vi "PIL_ICR.vi"(8 "error in (no error)":errorcluster, 10 "ICR Queue":refnum<queue>, 11 "UI Queue":refnum<queue>) -> (0 "error out":errorcluster)   [LabVIEW 2024]
uses:
  controls/QMH_ICR_Message.ctl
  controls/QMH_ICR_Command.ctl
  controls/QMH_UI_Message.ctl
  controls/QMH_UI_Command.ctl
  controls/HARDWARE_Resources.ctl
  controls/PROCESSING_Inputs.ctl
  controls/OPO_Inputs.ctl
  controls/QMH_ICR_Cluster.ctl
panel:
  out "RF Trap is ON":bool=TRUE caption="RF Trap"
  in  "OPO Inputs":T1={"OPO AutoAlignment ON"=FALSE, "OPO Start Value"=210.0, "OPO Stop Value"=270.0, "OPO Step"=10.0} {"OPO Step" min=1.0 max=60.0; "OPO Stop Value" min=210.0 max=270.0; "OPO Start Value" min=210.0 max=270.0}
  out "Number of  Loops":i16
  out "Loop":i16
  out "Number of Excitations":i16 caption="Excitations"
  out "PROCESSING  Inputs":T2={"Reference Mass"=300.0939, "Cyclotron Freq"=255.727, "Magnetron Freq"=0.001} caption="DATA Inputs" {"Magnetron Freq" format="%.5g"; "Cyclotron Freq" format="%.5g"; "Reference Mass" format="%.5g"}
  in  "Start":bool
  in  "Stop":bool
  in  "Send Trigger":bool
  out "Total Duration":i32
  out "Number of  Accumulations":i16
  out "Accumulation":i16
  in  "Use Software Trigger":bool=TRUE
  in  "Graph Chooser":T3(radio)=enum."Mass Spectrum"
  out "Remaining Time":string
  out "Spectrum Path":path
  out "Spectrum Prefix":string
  out "Spectrum Name":string
  out "Accum Name":string
  out "Mass Accumulated":cluster{dbl[], dbl[]}(graph)
  out "Mass Spectrum":cluster{dbl[], dbl[]}(graph)
  out "Frequency Spectrum":cluster{dbl[], dbl[]}(graph)
  out "Signal":cluster{dbl[], dbl[]}(graph)
  in  "HARDWARE Resources":T4={"AO6711 Physical Channels"="Analog/ao0:3", "AO6711 Task Name"="", "AO_6738 Physical Channels"="AO_6738/ao0:3", "AO6738 Task Name"="", "AWG5421 Resource Name"="Waveform", "DIGIT 5122 Resource Name"="Digitizer", "HSDIO Resource Name"="Sequencer"}
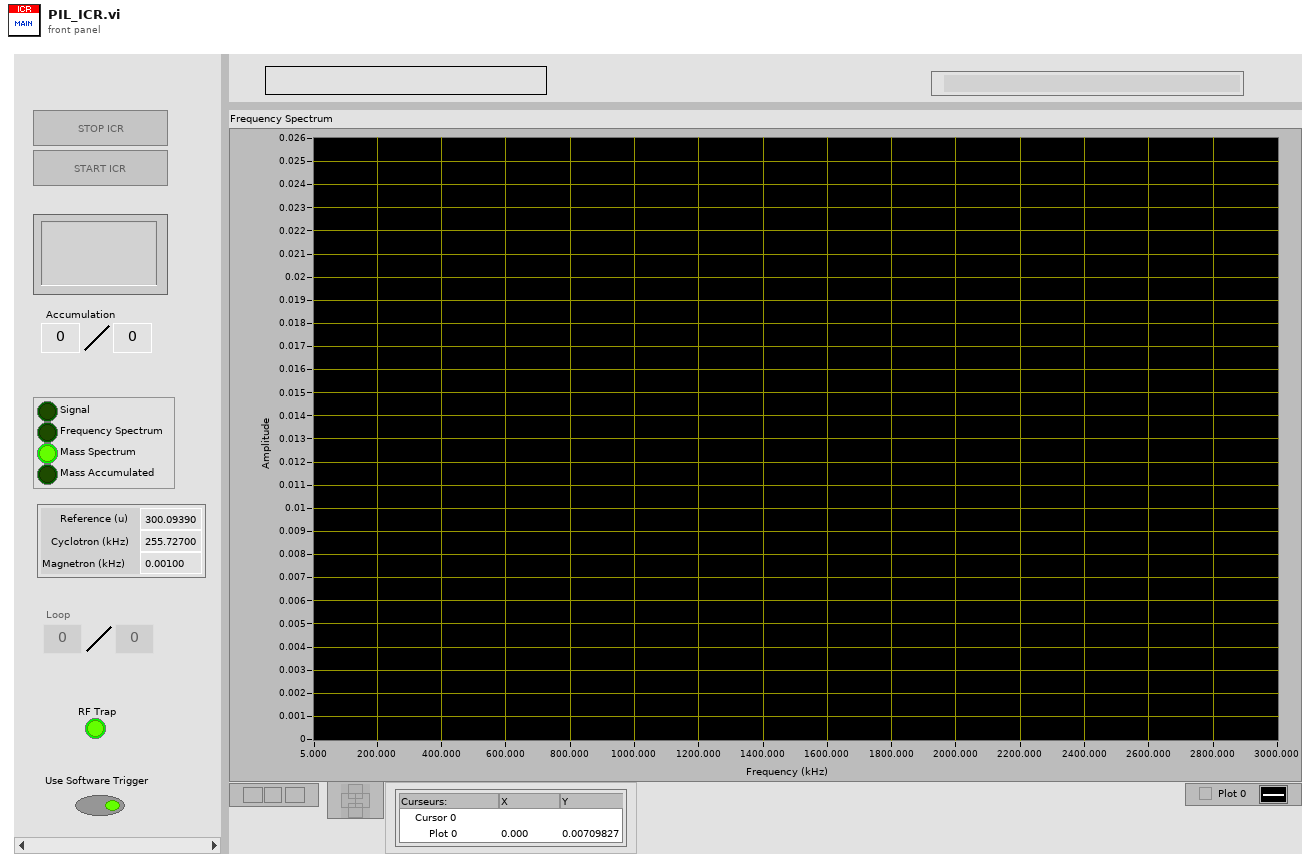
[diagram p1: front panel]
types:
  T1 = typedef "OPO_Inputs.ctl" = cluster{"OPO AutoAlignment ON":bool, "OPO Start Value":dbl, "OPO Stop Value":dbl, "OPO Step":dbl}
  T2 = typedef "PROCESSING_Inputs.ctl" = cluster{"Reference Mass":dbl, "Cyclotron Freq":dbl, "Magnetron Freq":dbl}
  T3 = enum32{"Signal", "Frequency Spectrum", "Mass Spectrum", "Mass Accumulated"}
  T4 = typedef "HARDWARE_Resources.ctl" = cluster{"AO6711 Physical Channels":tag, "AO6711 Task Name":refnum<k21>, "AO_6738 Physical Channels":tag, "AO6738 Task Name":refnum<k21>, "AWG5421 Resource Name":refnum<k15>, "DIGIT 5122 Resource Name":refnum<k15>, "HSDIO Resource Name":refnum<k15>}
  T5 = typedef "QMH_ICR_Cluster.ctl" = cluster{"Use Software Trigger":refnum<vi>, "Send Trigger":refnum<vi>, "Stop":refnum<vi>, "Start":refnum<vi>, "HARDWARE Resources":refnum<vi>, "Total Duration":refnum<vi>, "Remaining Time":refnum<vi>, "Accumulation":refnum<vi>, "Number of  Accumulations":refnum<vi>, "Number of  Excitations":refnum<vi>, "Graph Chooser":refnum<vi>, "Signal":refnum<vi>, "Frequency Spectrum":refnum<vi>, "Mass Spectrum":refnum<vi>, "Mass Accumulated":refnum<vi>, "Processing":refnum<vi>, "Spectrum Path":refnum<vi>, "Spectrum Prefix":refnum<vi>, "Spectrum Name":refnum<vi>, "Accum Name":refnum<vi>, "Disk Writing Done":refnum<notifier>, "Loop":refnum<vi>, "Number of Loops":refnum<vi>, "OPO Inputs":refnum<vi>, "RF Trap is ON":refnum<vi>}
  T6 = typedef "QMH_ICR_Command.ctl" = enum16{"Initialize", "Sequence Loop Setup", "Sequence Setup", "ICR Start", "ICR Stop", "Hardware Setup", "Next Sequence Loop", "Next Accumulation", "Waiting for Trigger", "Sequence Started", "Sequence Finished", "Sequence Loop Done", "Writing Data", "Hardware Reset", "Exit"}
  T7 = typedef "QMH_UI_Command.ctl" = enum16{"Initialize", "UI Load", "UI Save", "UI Save As", "UI Change Experiment", "UI Change Voltages", "UI Change Sequence", "UI Change Expert", "UI Change Loops", "UI Change Scientist", "Ready to Start", "UI Start", "Waiting for ICR", "UI Exit", "Update Experiment", "Update Report", "Update ICR Status", "Waiting for User"}
  T8 = typedef "QMH_ICR_Message.ctl" = cluster{"Command":T6, "Data":variant}
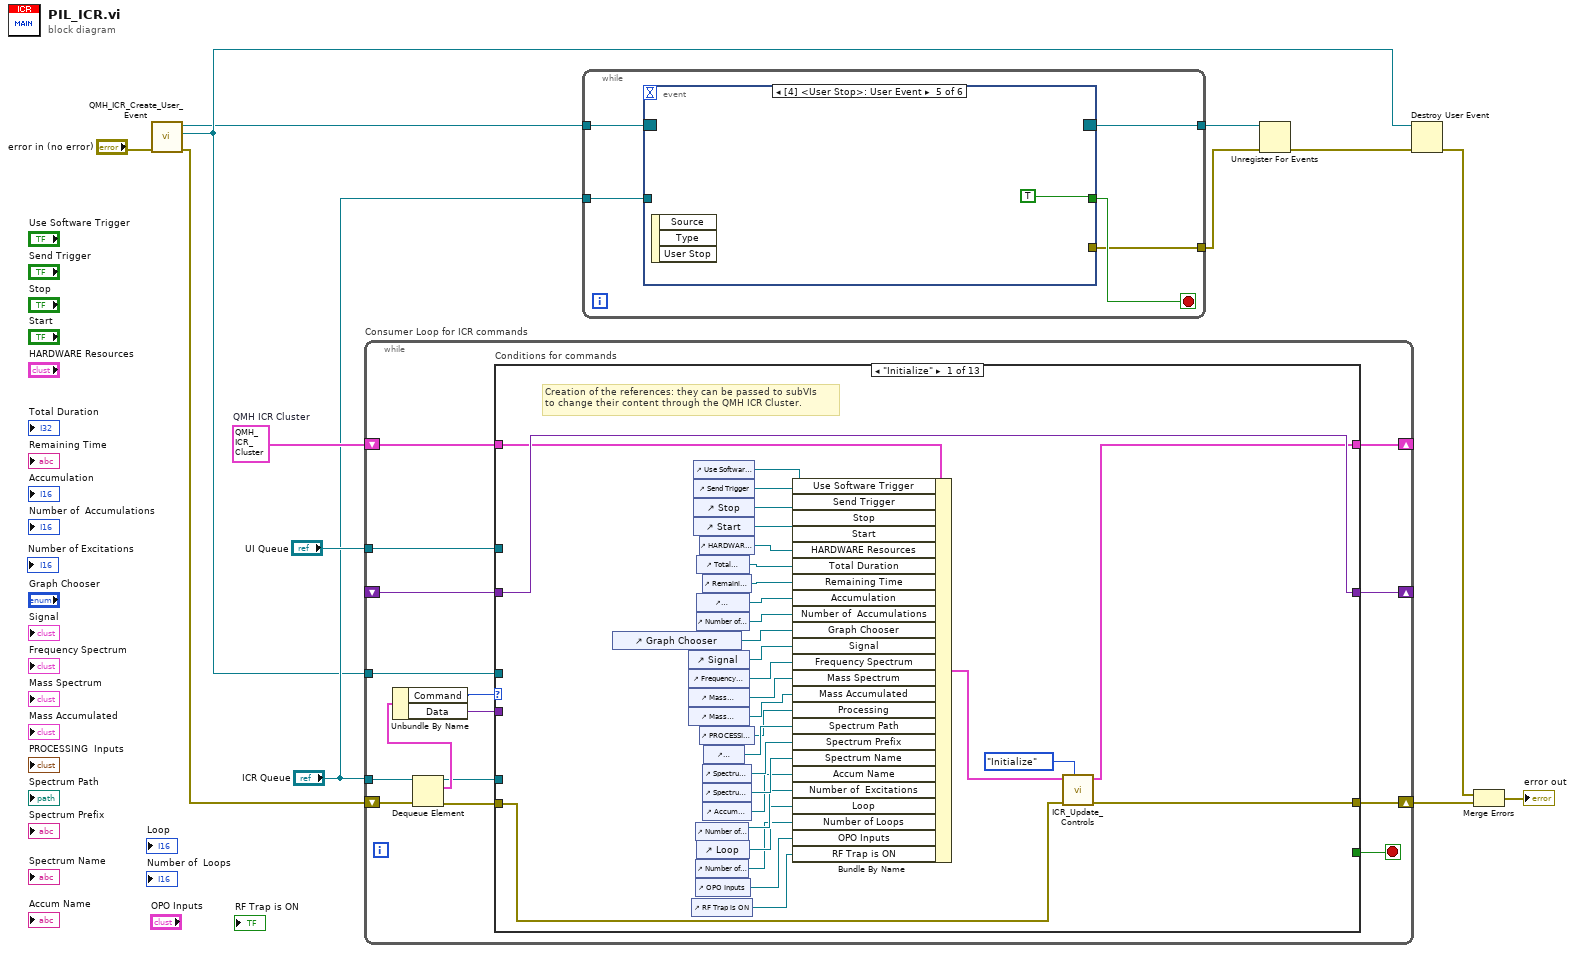
[diagram p0: block diagram]
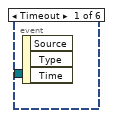
[diagram p2: hidden frame]
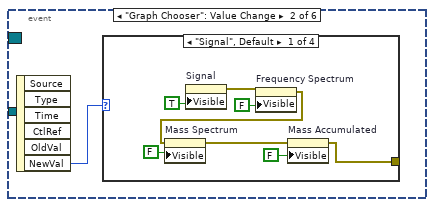
[diagram p3: hidden frame]
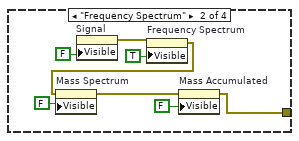
[diagram p4: hidden frame]
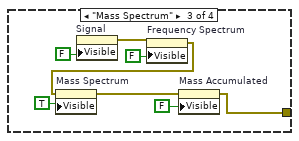
[diagram p5: hidden frame]
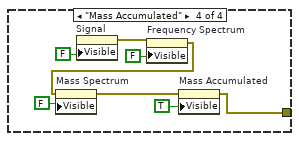
[diagram p6: hidden frame]
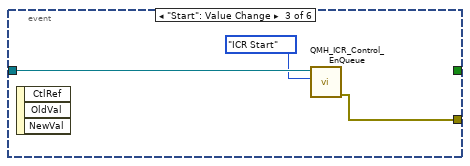
[diagram p7: hidden frame]
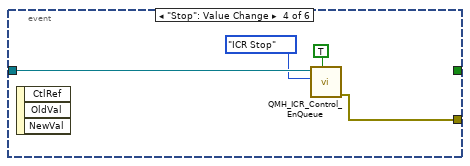
[diagram p8: hidden frame]
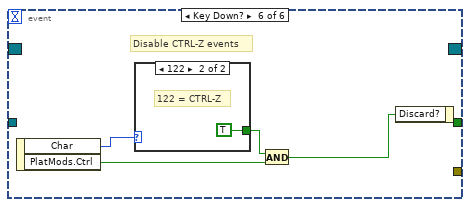
[diagram p9: hidden frame]
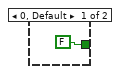
[diagram p10: hidden frame]
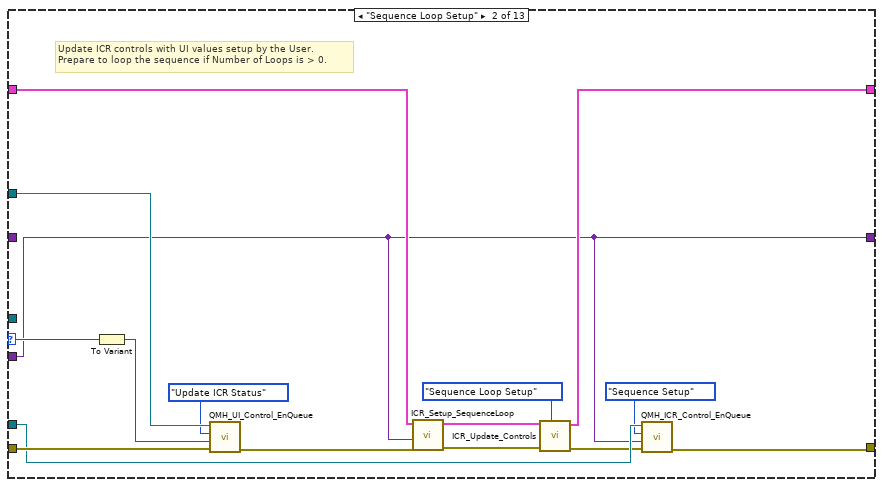
[diagram p11: hidden frame]
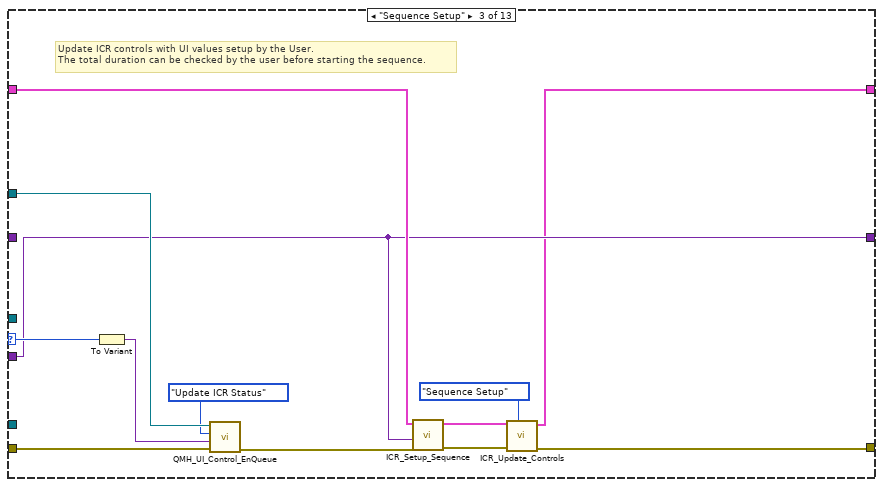
[diagram p12: hidden frame]
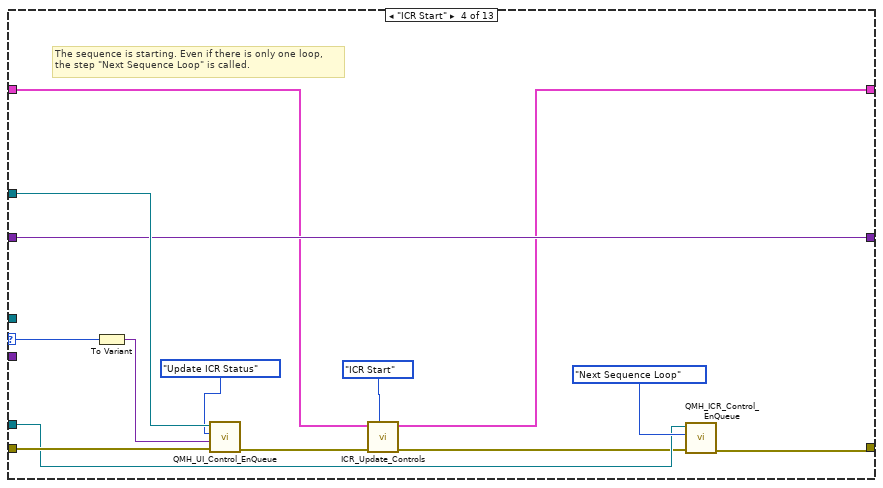
[diagram p13: hidden frame]
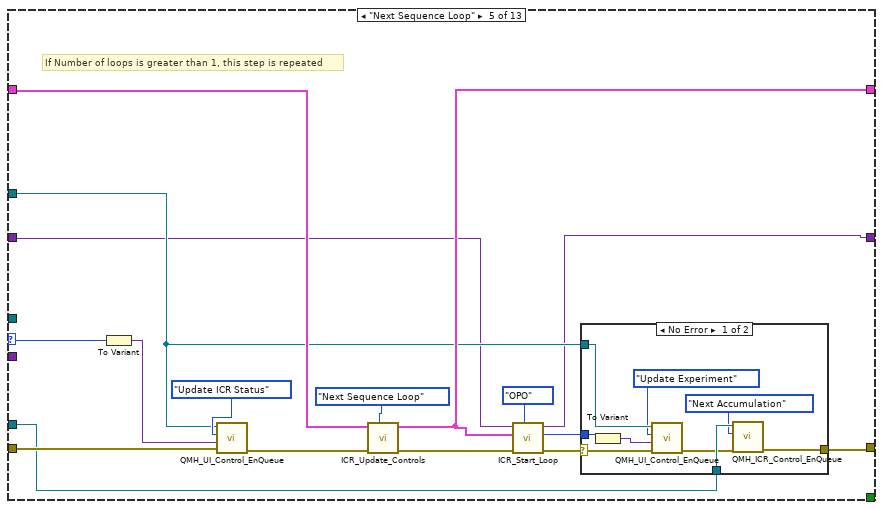
[diagram p14: hidden frame]
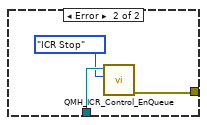
[diagram p15: hidden frame]
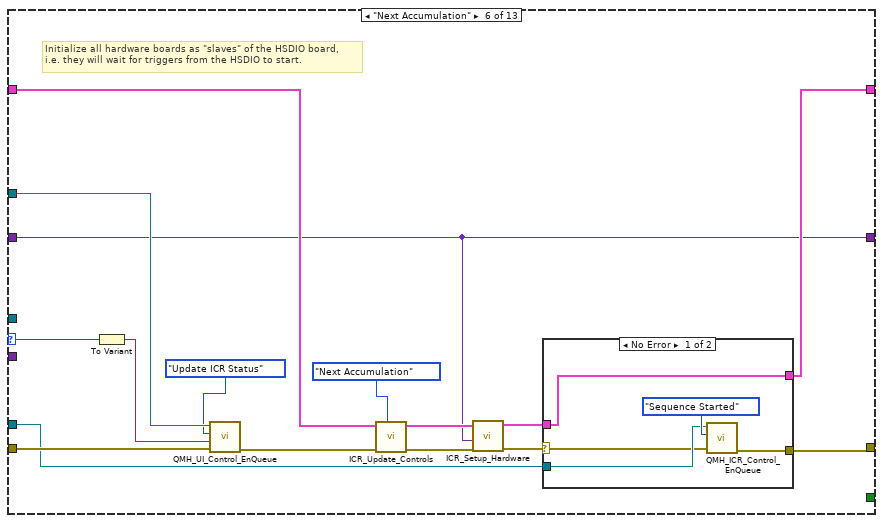
[diagram p16: hidden frame]
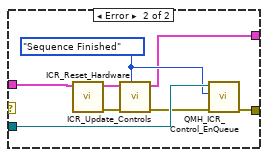
[diagram p17: hidden frame]
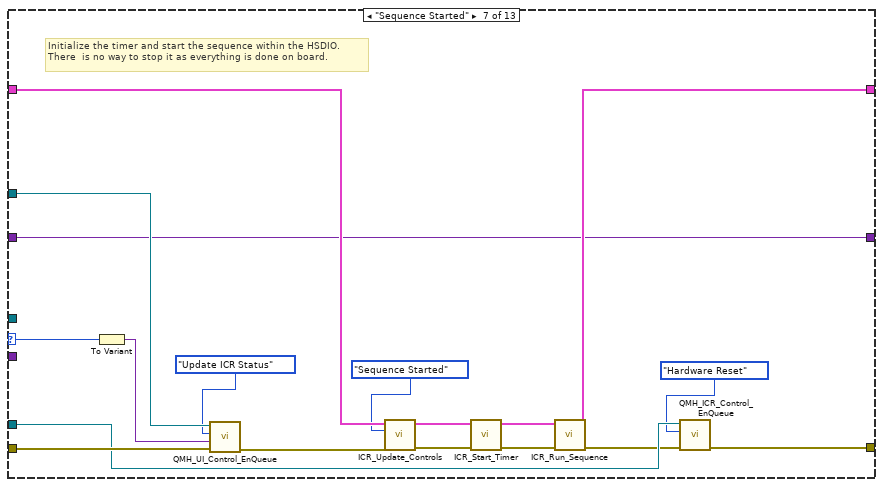
[diagram p18: hidden frame]
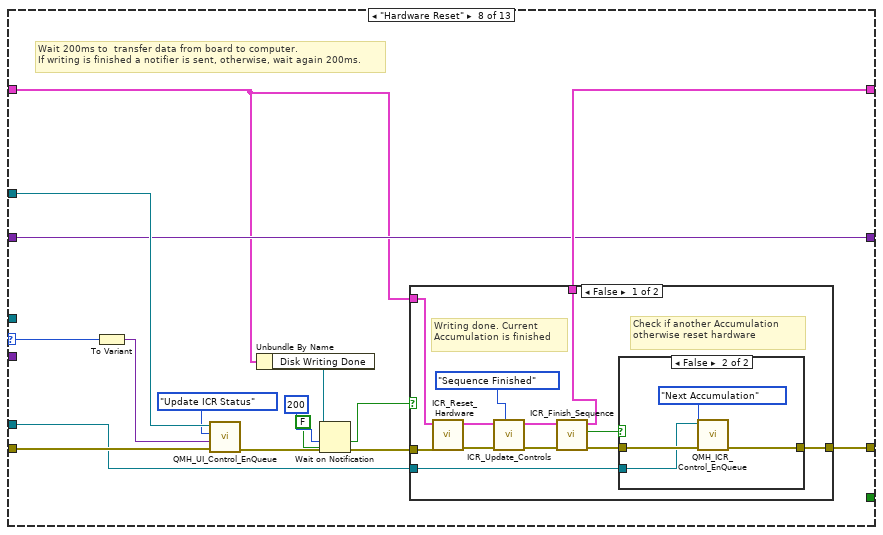
[diagram p19: hidden frame]
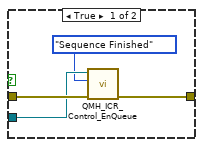
[diagram p20: hidden frame]
diagram:
  w6 = T5 {"Use Software Trigger"=refnum, "Send Trigger"=refnum, "Stop"=refnum, "Start"=refnum, "HARDWARE Resources"=refnum, "Total Duration"=refnum, "Remaining Time"=refnum, "Accumulation"=refnum, "Number of  Accumulations"=refnum, "Number of  Excitations"=refnum, "Graph Chooser"=refnum, "Signal"=refnum, "Frequency Spectrum"=refnum, "Mass Spectrum"=refnum, "Mass Accumulated"=refnum, "Processing"=refnum, "Spectrum Path"=refnum, "Spectrum Prefix"=refnum, "Spectrum Name"=refnum, "Accum Name"=refnum, "Disk Writing Done"=refnum, "Loop"=refnum, "Number of Loops"=refnum, "OPO Inputs"=refnum, "RF Trap is ON"=refnum}  # QMH ICR Cluster
  n1 = call "QMH_ICR_Create_User_Event.vi"("error in (no error)"="error in (no error)") -> ("error out"=w11:errorcluster, "User Stop Event"=w2:refnum<user-event>, "Refnum register for events"=w1:refnum<event-registration>)  [unwired: 8 in]
  n2 = while "Consumer Loop for ICR commands" {
    shift-right: [w19] -> w7
    shift-left: w11 -> [w26]
    tunnel: "ICR Queue" -> [w27]
    tunnel: "UI Queue" -> [w21]
    shift-right: [w18] -> _
    shift-left: _ -> [w17]
    tunnel: w2 -> [w16]
    shift-right: [w14] -> _
    shift-left: w6 -> [w15]
    stop <- w20 stop-if-true
    n3 = Dequeue Element(queue=w27, error in (no error)=w26) -> (queue out=w25:refnum<queue>, element=w28:T8, error out=w22:errorcluster)  [unwired: 2 out]
    n4 = Unbundle By Name(w28) -> ("Command"=w24:T6, "Data"=w23:variant)
    n5 = case "Conditions for commands" shown="\"Initialize\"" w24 {
      selector: w24 -> [_ w73 w86 w100 w114 w145 w176 w192 w234 w251 w277 _ _]
      tunnel: w25 -> [_ w64 _ w96 w111 w142 w173 w189 w228 w238 _ w287 _]
      tunnel: w23 -> [_ w60 w82 _ _ _ _ _ _ _ _ _ _]
      tunnel: w22 -> [w54 w72 w85 w99 w113 w144 w175 w191 w233 w250 w276 w279 _]
      tunnel: w21 -> [_ w74 w87 w101 w106 w146 w177 w193 w235 w252 w267 _ _]
      tunnel: [_ _ _ _ _ _ _ _ _ _ _ TRUE _] -> w20
      tunnel: [w52 w62 w77 w97 w116 w143 w174 w190 w230 w247 w275 w280 _] -> w19
      tunnel: [w59 w60 w82 w95 w104 w132 w169 w187 w232 w237 w274 _ _] -> w18
      tunnel: w17 -> [w59 _ _ w95 w105 w132 w169 w187 w232 w237 w274 _ _]
      tunnel: w16 -> [_ _ _ _ _ _ _ _ _ _ _ w284 _]
      tunnel: w15 -> [w51 w70 w83 w93 w112 w139 w172 w186 w225 w242 w272 _ _]
      tunnel: [w53 w67 w79 w92 w108 w135 w170 w188 w223 w244 w270 _ _] -> w14
      frame "Initialize" {
        # "Creation of the references: they can be passed to subVIs\nto change their content through the QMH ICR Cluster."
        n6 = control-ref of="Graph Chooser"() -> (w55:refnum<vi>)
        n7 = control-ref of="Signal"() -> (w34:refnum<vi>)
        n8 = control-ref of="Frequency Spectrum"() -> (w56:refnum<vi>)
        n9 = control-ref of="Mass Spectrum"() -> (w57:refnum<vi>)
        n10 = control-ref of="Mass Accumulated"() -> (w45:refnum<vi>)
        n11 = control-ref of="RF Trap is ON"() -> (w29:refnum<vi>)
        n12 = control-ref of="Use Software Trigger"() -> (w58:refnum<vi>)
        n13 = control-ref of="Send Trigger"() -> (w43:refnum<vi>)
        n14 = control-ref of="Stop"() -> (w42:refnum<vi>)
        n15 = control-ref of="Start"() -> (w41:refnum<vi>)
        n16 = control-ref of="Number of Excitations"() -> (w33:refnum<vi>)
        n17 = control-ref of="Number of  Loops"() -> (w31:refnum<vi>)
        n18 = control-ref of="OPO Inputs"() -> (w30:refnum<vi>)
        n19 = control-ref of="Total Duration"() -> (w39:refnum<vi>)
        n20 = control-ref of="Accumulation"() -> (w36:refnum<vi>)
        n21 = control-ref of="Number of  Accumulations"() -> (w35:refnum<vi>)
        n22 = control-ref of="Loop"() -> (w32:refnum<vi>)
        n23 = control-ref of="HARDWARE Resources"() -> (w40:refnum<vi>)
        n24 = control-ref of="PROCESSING  Inputs"() -> (w44:refnum<vi>)
        n25 = control-ref of="Remaining Time"() -> (w38:refnum<vi>)
        n26 = control-ref of="Spectrum Prefix"() -> (w47:refnum<vi>)
        n27 = control-ref of="Spectrum Name"() -> (w46:refnum<vi>)
        n28 = control-ref of="Accum Name"() -> (w37:refnum<vi>)
        n29 = control-ref of="Spectrum Path"() -> (w48:refnum<vi>)
        n30 = Bundle By Name(cluster=w51, "Use Software Trigger"=w58, "Send Trigger"=w43, "Stop"=w42, "Start"=w41, "HARDWARE Resources"=w40, "Total Duration"=w39, "Remaining Time"=w38, "Accumulation"=w36, "Number of  Accumulations"=w35, "Graph Chooser"=w55, "Signal"=w34, "Frequency Spectrum"=w56, "Mass Spectrum"=w57, "Mass Accumulated"=w45, "Processing"=w44, "Spectrum Path"=w48, "Spectrum Prefix"=w47, "Spectrum Name"=w46, "Accum Name"=w37, "Number of  Excitations"=w33, "Loop"=w32, "Number of Loops"=w31, "OPO Inputs"=w30, "RF Trap is ON"=w29) -> (w50:T5)
        n31 = call "ICR_Update_Controls.vi"("Command"=QMH_ICR_Command."Initialize", "error in (no error)"=w54, "QMH ICR Cluster"=w50) -> ("error out"=w52:errorcluster, "QMH ICR Cluster"=w53:T5)  [unwired: 7 in]
      }
      frame "Sequence Loop Setup" {
        # "Update ICR controls with UI values setup by the User.\nPrepare to loop the sequence if Number of Loops is > 0."
        n32 = To Variant(anything=w73) -> (Variant=w75:variant)
        n33 = call "QMH_UI_Control_EnQueue.vi"("error in (no error)"=w72, "Variant"=w75, "Command"=QMH_UI_Command."Update ICR Status", "UI Queue"=w74) -> ("error out"=w71:errorcluster)  [unwired: 6 in, 1 out]
        n34 = call "ICR_Setup_SequenceLoop.vi"("error in (no error)"=w71, "QMH UI Cluster"=w60, "QMH ICR Cluster"=w70) -> ("error out"=w69:errorcluster, "QMH ICR Cluster"=w68:T5)  [unwired: 7 in]
        n35 = call "ICR_Update_Controls.vi"("Command"=QMH_ICR_Command."Sequence Loop Setup", "error in (no error)"=w69, "QMH ICR Cluster"=w68) -> ("error out"=w63:errorcluster, "QMH ICR Cluster"=w67:T5)  [unwired: 7 in]
        n36 = call "QMH_ICR_Control_EnQueue.vi"("error in (no error)"=w63, "Variant"=w60, "Command"=QMH_ICR_Command."Sequence Setup", "ICR Queue"=w64) -> ("error out"=w62:errorcluster)  [unwired: 6 in, 1 out]
      }
      frame "Sequence Setup" {
        # "Update ICR controls with UI values setup by the User.\nThe total duration can be checked by the user before starting the sequence."
        n37 = To Variant(anything=w86) -> (Variant=w88:variant)
        n38 = call "QMH_UI_Control_EnQueue.vi"("error in (no error)"=w85, "Variant"=w88, "Command"=QMH_UI_Command."Update ICR Status", "UI Queue"=w87) -> ("error out"=w84:errorcluster)  [unwired: 6 in, 1 out]
        n39 = call "ICR_Setup_Sequence.vi"("error in (no error)"=w84, "QMH UI Cluster"=w82, "QMH ICR Cluster"=w83) -> ("error out"=w81:errorcluster, "QMH ICR Cluster"=w80:T5)  [unwired: 7 in]
        n40 = call "ICR_Update_Controls.vi"("Command"=QMH_ICR_Command."Sequence Setup", "error in (no error)"=w81, "QMH ICR Cluster"=w80) -> ("error out"=w77:errorcluster, "QMH ICR Cluster"=w79:T5)  [unwired: 7 in]
      }
      frame "ICR Start" {
        # "The sequence is starting. Even if there is only one loop,\nthe step \"Next Sequence Loop\" is called."
        n41 = To Variant(anything=w100) -> (Variant=w102:variant)
        n42 = call "QMH_UI_Control_EnQueue.vi"("error in (no error)"=w99, "Variant"=w102, "Command"=QMH_UI_Command."Update ICR Status", "UI Queue"=w101) -> ("error out"=w89:errorcluster)  [unwired: 6 in, 1 out]
        n43 = call "ICR_Update_Controls.vi"("Command"=QMH_ICR_Command."ICR Start", "error in (no error)"=w89, "QMH ICR Cluster"=w93) -> ("error out"=w90:errorcluster, "QMH ICR Cluster"=w92:T5)  [unwired: 7 in]
        n44 = call "QMH_ICR_Control_EnQueue.vi"("error in (no error)"=w90, "Command"=QMH_ICR_Command."Next Sequence Loop", "ICR Queue"=w96) -> ("error out"=w97:errorcluster)  [unwired: 7 in, 1 out]
      }
      frame "Next Sequence Loop" {
        # "If Number of loops is greater than 1, this step is repeated"
        n45 = To Variant(anything=w114) -> (Variant=w119:variant)
        n46 = call "QMH_UI_Control_EnQueue.vi"("error in (no error)"=w113, "Variant"=w119, "Command"=QMH_UI_Command."Update ICR Status", "UI Queue"=w106) -> ("error out"=w118:errorcluster)  [unwired: 6 in, 1 out]
        n47 = call "ICR_Update_Controls.vi"("Command"=QMH_ICR_Command."Next Sequence Loop", "error in (no error)"=w118, "QMH ICR Cluster"=w112) -> ("error out"=w110:errorcluster, "QMH ICR Cluster"=w108:T5)  [unwired: 7 in]
        n48 = call "ICR_Start_Loop.vi"("Loop Selector"=enum16{"OPO", "Other"}."OPO", "error in (no error)"=w110, "QMH ICR Cluster"=w108, "QMH UI Cluster"=w105) -> ("error out"=w103:errorcluster, "Loop Current Value"=w107:i16, "QMH UI Cluster Output"=w104:variant)  [unwired: 5 in]
        n49 = case shown="No Error" w103 {
          selector: w103 -> [w120 _]
          tunnel: [w128 w131] -> w116
          tunnel: w111 -> [w127 w130]
          tunnel: w107 -> [w124 _]
          tunnel: w106 -> [w122 _]
          frame No Error {
            n50 = To Variant(anything=w124) -> (Variant=w123:variant)
            n51 = call "QMH_UI_Control_EnQueue.vi"("error in (no error)"=w120, "Variant"=w123, "Command"=QMH_UI_Command."Update Experiment", "UI Queue"=w122) -> ("error out"=w125:errorcluster)  [unwired: 6 in, 1 out]
            n52 = call "QMH_ICR_Control_EnQueue.vi"("error in (no error)"=w125, "Command"=QMH_ICR_Command."Next Accumulation", "ICR Queue"=w127) -> ("error out"=w128:errorcluster)  [unwired: 7 in, 1 out]
          }
          frame Error {
            n53 = call "QMH_ICR_Control_EnQueue.vi"("Command"=QMH_ICR_Command."ICR Stop", "ICR Queue"=w130) -> ("error out"=w131:errorcluster)  [unwired: 8 in, 1 out]
          }
        }
      }
      frame "Next Accumulation" {
        # "Initialize all hardware boards as \"slaves\" of the HSDIO board,\ni.e. they will wait for triggers from the HSDIO to start."
        n54 = To Variant(anything=w145) -> (Variant=w147:variant)
        n55 = call "QMH_UI_Control_EnQueue.vi"("error in (no error)"=w144, "Variant"=w147, "Command"=QMH_UI_Command."Update ICR Status", "UI Queue"=w146) -> ("error out"=w141:errorcluster)  [unwired: 6 in, 1 out]
        n56 = call "ICR_Update_Controls.vi"("Command"=QMH_ICR_Command."Next Accumulation", "error in (no error)"=w141, "QMH ICR Cluster"=w139) -> ("error out"=w140:errorcluster, "QMH ICR Cluster"=w138:T5)  [unwired: 7 in]
        n57 = call "ICR_Setup_Hardware.vi"("error in (no error)"=w140, "QMH UI Cluster"=w132, "QMH ICR Cluster"=w138) -> ("error out"=w134:errorcluster, "QMH ICR Cluster"=w137:T5)  [unwired: 7 in]
        n58 = case shown="No Error" w134 {
          selector: w134 -> [w148 _]
          tunnel: [w151 w156] -> w143
          tunnel: w142 -> [w150 w158]
          tunnel: w137 -> [w149 w154]
          tunnel: [w149 w153] -> w135
          frame No Error {
            n59 = call "QMH_ICR_Control_EnQueue.vi"("error in (no error)"=w148, "Command"=QMH_ICR_Command."Sequence Started", "ICR Queue"=w150) -> ("error out"=w151:errorcluster)  [unwired: 7 in, 1 out]
          }
          frame Error {
            w155 = QMH_ICR_Command."Sequence Finished" ("Command")
            n60 = call "ICR_Reset_Hardware.vi"("QMH ICR Cluster"=w154) -> ("error out"=w159:errorcluster, "QMH ICR Cluster"=w160:T5)  [unwired: 9 in]
            n61 = call "ICR_Update_Controls.vi"("Command"=w155, "error in (no error)"=w159, "QMH ICR Cluster"=w160) -> ("error out"=w157:errorcluster, "QMH ICR Cluster"=w153:T5)  [unwired: 7 in]
            n62 = call "QMH_ICR_Control_EnQueue.vi"("error in (no error)"=w157, "Command"=w155, "ICR Queue"=w158) -> ("error out"=w156:errorcluster)  [unwired: 7 in, 1 out]
          }
        }
      }
      frame "Sequence Started" {
        # "Initialize the timer and start the sequence within the HSDIO. \nThere  is no way to stop it as everything is done on board."
        n63 = To Variant(anything=w176) -> (Variant=w178:variant)
        n64 = call "QMH_UI_Control_EnQueue.vi"("error in (no error)"=w175, "Variant"=w178, "Command"=QMH_UI_Command."Update ICR Status", "UI Queue"=w177) -> ("error out"=w166:errorcluster)  [unwired: 6 in, 1 out]
        n65 = call "ICR_Update_Controls.vi"("Command"=QMH_ICR_Command."Sequence Started", "error in (no error)"=w166, "QMH ICR Cluster"=w172) -> ("error out"=w163:errorcluster, "QMH ICR Cluster"=w167:T5)  [unwired: 7 in]
        n66 = call "ICR_Start_Timer.vi"("error in (no error)"=w163, "QMH ICR Cluster"=w167) -> ("error out"=w162:errorcluster, "QMH ICR Cluster"=w164:T5)  [unwired: 8 in]
        n67 = call "ICR_Run_Sequence.vi"("error in (no error)"=w162, "QMH ICR Cluster"=w164) -> ("error out"=w171:errorcluster, "QMH ICR Cluster"=w170:T5)  [unwired: 8 in]
        n68 = call "QMH_ICR_Control_EnQueue.vi"("error in (no error)"=w171, "Command"=QMH_ICR_Command."Hardware Reset", "ICR Queue"=w173) -> ("error out"=w174:errorcluster)  [unwired: 7 in, 1 out]
      }
      frame "Hardware Reset" {
        # "Wait 200ms to  transfer data from board to computer.\nIf writing is finished a notifier is sent, otherwise, wait again 200ms."
        n69 = To Variant(anything=w192) -> (Variant=w194:variant)
        n70 = call "QMH_UI_Control_EnQueue.vi"("error in (no error)"=w191, "Variant"=w194, "Command"=QMH_UI_Command."Update ICR Status", "UI Queue"=w193) -> ("error out"=w183:errorcluster)  [unwired: 6 in, 1 out]
        n71 = Unbundle By Name(w186) -> ("Disk Writing Done"=w185:refnum<notifier>)
        n72 = Wait on Notification(notifier=w185, ignore previous (F)=FALSE ("ignorer les précédents (F)"), timeout in ms (-1)=200 ("timeout en ms (-1)"), error in (no error)=w183) -> (timed out?=w181:bool, error out=w182:errorcluster)  [unwired: 2 out]
        n73 = case shown="False" w181 {
          tunnel: [w206 w220] -> w190
          tunnel: w189 -> [w205 w221]
          tunnel: [w203 w216] -> w188
          tunnel: w186 -> [w196 w217]
          tunnel: w182 -> [w195 w219]
          frame False {
            # "Check if another Accumulation\notherwise reset hardware"
            # "Writing done. Current \nAccumulation is finished"
            n74 = call "ICR_Reset_Hardware.vi"("error in (no error)"=w195, "QMH ICR Cluster"=w196) -> ("error out"=w199:errorcluster, "QMH ICR Cluster"=w201:T5)  [unwired: 8 in]
            n75 = call "ICR_Update_Controls.vi"("Command"=QMH_ICR_Command."Sequence Finished", "error in (no error)"=w199, "QMH ICR Cluster"=w201) -> ("error out"=w198:errorcluster, "QMH ICR Cluster"=w200:T5)  [unwired: 7 in]
            n76 = call "ICR_Finish_Sequence.vi"("error in (no error)"=w198, "QMH ICR Cluster"=w200) -> ("error out"=w204:errorcluster, "Is Finished ?"=w202:bool, "QMH ICR Cluster"=w203:T5)  [unwired: 7 in]
            n77 = case shown="False" w202 {
              tunnel: w204 -> [w210 w214]
              tunnel: [w209 w213] -> w206
              tunnel: w205 -> [w208 w212]
              frame True {
                n78 = call "QMH_ICR_Control_EnQueue.vi"("error in (no error)"=w210, "Command"=QMH_ICR_Command."Sequence Finished", "ICR Queue"=w208) -> ("error out"=w209:errorcluster)  [unwired: 7 in, 1 out]
              }
              frame False {
                n79 = call "QMH_ICR_Control_EnQueue.vi"("error in (no error)"=w214, "Command"=QMH_ICR_Command."Next Accumulation", "ICR Queue"=w212) -> ("error out"=w213:errorcluster)  [unwired: 7 in, 1 out]
              }
            }
          }
          frame True {
            # "Writing not done. Wait again by sending\nthe same message  to the ICR Queue"
            n80 = call "ICR_Update_Controls.vi"("Command"=QMH_ICR_Command."Hardware Reset", "error in (no error)"=w219, "QMH ICR Cluster"=w217) -> ("error out"=w218:errorcluster, "QMH ICR Cluster"=w216:T5)  [unwired: 7 in]
            n81 = call "QMH_ICR_Control_EnQueue.vi"("error in (no error)"=w218, "Command"=QMH_ICR_Command."Hardware Reset", "ICR Queue"=w221) -> ("error out"=w220:errorcluster)  [unwired: 7 in, 1 out]
          }
        }
      }
      frame "Sequence Finished" {
        n82 = To Variant(anything=w234) -> (Variant=w236:variant)
        n83 = call "QMH_UI_Control_EnQueue.vi"("error in (no error)"=w233, "Variant"=w236, "Command"=QMH_UI_Command."Update ICR Status", "UI Queue"=w235) -> ("error out"=w231:errorcluster)  [unwired: 6 in, 1 out]
        n84 = call "ICR_Update_Controls.vi"("Command"=QMH_ICR_Command."Sequence Finished", "error in (no error)"=w231, "QMH ICR Cluster"=w225) -> ("error out"=w226:errorcluster, "QMH ICR Cluster"=w223:T5)  [unwired: 7 in]
        n85 = call "QMH_ICR_Control_EnQueue.vi"("error in (no error)"=w226, "Command"=QMH_ICR_Command."Sequence Loop Done", "ICR Queue"=w228) -> ("error out"=w230:errorcluster)  [unwired: 7 in, 1 out]
      }
      frame "Sequence Loop Done" {
        n86 = To Variant(anything=w251) -> (Variant=w253:variant)
        n87 = call "QMH_UI_Control_EnQueue.vi"("error in (no error)"=w250, "Variant"=w253, "Command"=QMH_UI_Command."Update ICR Status", "UI Queue"=w252) -> ("error out"=w249:errorcluster, "UI Queue"=w248:refnum<queue>)  [unwired: 6 in]
        n88 = call "ICR_Update_Controls.vi"("Command"=QMH_ICR_Command."Sequence Loop Done", "error in (no error)"=w249, "QMH ICR Cluster"=w242) -> ("error out"=w243:errorcluster, "QMH ICR Cluster"=w241:T5)  [unwired: 7 in]
        n89 = call "ICR_Finish_SequenceLoop.vi"("error in (no error)"=w243, "QMH ICR Cluster"=w241) -> ("error out"=w245:errorcluster, "Is Finished ?"=w239:bool, "QMH ICR Cluster"=w244:T5)  [unwired: 7 in]
        n90 = case shown="False" w239 {
          tunnel: w248 -> [_ w265]
          tunnel: [w257 w263] -> w247
          tunnel: w245 -> [w254 w262]
          tunnel: w238 -> [w260 _]
          tunnel: w237 -> [w258 _]
          frame False {
            n91 = call "QMH_ICR_Control_EnQueue.vi"("error in (no error)"=w254, "Variant"=w258, "Command"=QMH_ICR_Command."Sequence Setup", "ICR Queue"=w260) -> ("error out"=w261:errorcluster, "ICR Queue"=w256:refnum<queue>)  [unwired: 6 in]
            n92 = call "QMH_ICR_Control_EnQueue.vi"("error in (no error)"=w261, "Command"=QMH_ICR_Command."ICR Start", "ICR Queue"=w256) -> ("error out"=w257:errorcluster)  [unwired: 7 in, 1 out]
          }
          frame True {
            n93 = call "QMH_UI_Control_EnQueue.vi"("error in (no error)"=w262, "Command"=QMH_UI_Command."Ready to Start", "UI Queue"=w265) -> ("error out"=w263:errorcluster)  [unwired: 7 in, 1 out]
          }
        }
      }
      frame "ICR Stop" {
        n94 = To Variant(anything=w277) -> (Variant=w278:variant)
        n95 = call "QMH_UI_Control_EnQueue.vi"("error in (no error)"=w276, "Variant"=w278, "Command"=QMH_UI_Command."Update ICR Status", "UI Queue"=w267) -> ("error out"=w271:errorcluster)  [unwired: 6 in, 1 out]
        n96 = call "ICR_Update_Controls.vi"("Command"=QMH_ICR_Command."ICR Stop", "error in (no error)"=w271, "QMH ICR Cluster"=w272) -> ("error out"=w269:errorcluster, "QMH ICR Cluster"=w270:T5)  [unwired: 7 in]
        n97 = call "QMH_UI_Control_EnQueue.vi"("error in (no error)"=w269, "Command"=QMH_UI_Command."Ready to Start", "UI Queue"=w267) -> ("error out"=w275:errorcluster)  [unwired: 7 in, 1 out]
      }
      frame "Exit" {
        n98 = One Button Dialog(message="Software should stop") -> ()  [unwired: 1 in, 1 out]
        n99 = Generate User Event(user event=w284, event data cluster=TRUE ("données d'événement")) -> (error out=w282:errorcluster)  [unwired: 2 in, 1 out]
        n100 = Release Queue(queue=w287, error in (no error)=w279) -> (error out=w281:errorcluster)  [unwired: 1 in, 2 out]
        n101 = Merge Errors(w282, w281) -> (w280:errorcluster)
      }
      frame Default {
        # "Left empty to force to wire all conditions.\nThis condition should never happen."
      }
    }
  }
  n102 = while {
    tunnel: [w291] -> w10
    tunnel: [w290] -> w9
    tunnel: "ICR Queue" -> [w289]
    tunnel: w1 -> [w288]
    stop <- w292 stop-if-true
    n103 = event shown="[4] <User Stop>: User Event" {
      selector: w288 -> [_ _ _ _ _ _]
      dyn-events: [_ _ _ _ _ _] -> w291
      timeout: _ -> [_ _ _ _ _ _]
      tunnel: [_ _ _ _ TRUE _] -> w292
      tunnel: [_ _ w328 w332 _ _] -> w290
      tunnel: w289 -> [_ _ w327 w331 _ _]
      event Timeout {
        n104 = event-data() -> ()  [unwired: 1 in, 3 out]
      }
      event "Graph Chooser": Value Change {
        n105 = event-data() -> ("NewVal"=w293:T3)  [unwired: 1 in, 5 out]
        n106 = case shown="\"Signal\", Default" w293 {
          tunnel: [w294 w305 w313 w318] -> _
          frame "Signal", Default {
            n107 = property on="Signal" class="XYGraph (strict)"("Visible"=TRUE) -> (error out=w297:errorcluster)  [unwired: 2 in, 1 out]
            n108 = property on="Frequency Spectrum" class="XYGraph (strict)"(error in=w297, "Visible"=FALSE) -> (error out=w296:errorcluster)  [unwired: 1 in, 1 out]
            n109 = property on="Mass Spectrum" class="XYGraph (strict)"(error in=w296, "Visible"=FALSE) -> (error out=w295:errorcluster)  [unwired: 1 in, 1 out]
            n110 = property on="Mass Accumulated" class="XYGraph (strict)"(error in=w295, "Visible"=FALSE) -> (error out=w294:errorcluster)  [unwired: 1 in, 1 out]
          }
          frame "Frequency Spectrum" {
            n111 = property on="Signal" class="XYGraph (strict)"("Visible"=FALSE) -> (error out=w302:errorcluster)  [unwired: 2 in, 1 out]
            n112 = property on="Frequency Spectrum" class="XYGraph (strict)"(error in=w302, "Visible"=TRUE) -> (error out=w303:errorcluster)  [unwired: 1 in, 1 out]
            n113 = property on="Mass Spectrum" class="XYGraph (strict)"(error in=w303, "Visible"=FALSE) -> (error out=w304:errorcluster)  [unwired: 1 in, 1 out]
            n114 = property on="Mass Accumulated" class="XYGraph (strict)"(error in=w304, "Visible"=FALSE) -> (error out=w305:errorcluster)  [unwired: 1 in, 1 out]
          }
          frame "Mass Spectrum" {
            n115 = property on="Signal" class="XYGraph (strict)"("Visible"=FALSE) -> (error out=w310:errorcluster)  [unwired: 2 in, 1 out]
            n116 = property on="Frequency Spectrum" class="XYGraph (strict)"(error in=w310, "Visible"=FALSE) -> (error out=w311:errorcluster)  [unwired: 1 in, 1 out]
            n117 = property on="Mass Spectrum" class="XYGraph (strict)"(error in=w311, "Visible"=TRUE) -> (error out=w312:errorcluster)  [unwired: 1 in, 1 out]
            n118 = property on="Mass Accumulated" class="XYGraph (strict)"(error in=w312, "Visible"=FALSE) -> (error out=w313:errorcluster)  [unwired: 1 in, 1 out]
          }
          frame "Mass Accumulated" {
            n119 = property on="Signal" class="XYGraph (strict)"("Visible"=FALSE) -> (error out=w321:errorcluster)  [unwired: 2 in, 1 out]
            n120 = property on="Frequency Spectrum" class="XYGraph (strict)"(error in=w321, "Visible"=FALSE) -> (error out=w320:errorcluster)  [unwired: 1 in, 1 out]
            n121 = property on="Mass Spectrum" class="XYGraph (strict)"(error in=w320, "Visible"=FALSE) -> (error out=w319:errorcluster)  [unwired: 1 in, 1 out]
            n122 = property on="Mass Accumulated" class="XYGraph (strict)"(error in=w319, "Visible"=TRUE) -> (error out=w318:errorcluster)  [unwired: 1 in, 1 out]
          }
        }
      }
      event "Start": Value Change {
        n123 = event-data() -> ()  [unwired: 1 in, 3 out]
        n124 = call "QMH_ICR_Control_EnQueue.vi"("Command"=QMH_ICR_Command."ICR Start", "ICR Queue"=w327) -> ("error out"=w328:errorcluster)  [unwired: 8 in, 1 out]
      }
      event "Stop": Value Change {
        n125 = event-data() -> ()  [unwired: 1 in, 3 out]
        n126 = call "QMH_ICR_Control_EnQueue.vi"("Last ?"=TRUE, "Command"=QMH_ICR_Command."ICR Stop", "ICR Queue"=w331) -> ("error out"=w332:errorcluster)  [unwired: 7 in, 1 out]
      }
      event User Event {
        n127 = event-data() -> ()  [unwired: 1 in, 3 out]
      }
      event Key Down? {
        # "Disable CTRL-Z events"
        n128 = event-data() -> ("Char"=w337:i16, "PlatMods.Ctrl"=w335:bool)  [unwired: 1 in]
        n129 = case shown="122" w337 {
          tunnel: [FALSE TRUE] -> w336
          frame 0, Default {
          }
          frame 122 {
            # "122 = CTRL-Z"
          }
        }
        n130 = And(x=w336, y=w335) -> (x .and. y?=w334:bool)
        n131 = event-data("Discard?"=w334) -> ()  [unwired: 1 in, 1 out]
      }
    }
  }
  n132 = Unregister For Events(event registration refnum=w10, error in=w9) -> (error out=w4:errorcluster)
  n133 = Destroy User Event(user event=w2, error in=w4) -> (error out=w3:errorcluster)
  n134 = Merge Errors(w3, w7) -> (→"error out":errorcluster)
